vi "Controller - Fire Command.vi"(8 "error in (no error)":errorcluster, 9 "Data":variant, 10 "CMD":T1, 11 "View Model":T2) -> (0 "error out":errorcluster)   [LabVIEW 2017]
doc: "Generate command with parameters to Controller"
uses:
  View Model/Controls/View Model.ctl
  View Model/Controls/Shared Model.ctl
  Error Handler/Controls/Error Model.ctl
  Error Handler/Controls/Error Event.ctl
  Error Handler/Controls/Error Type.ctl
  Controls/Controller Model.ctl
  Controls/Controller Event.ctl
  Controls/Controller Command.ctl
  Controls/Controller Overhead.ctl
  Real-Time/RT Status.ctl
  Real-Time/RT Loop Status.ctl
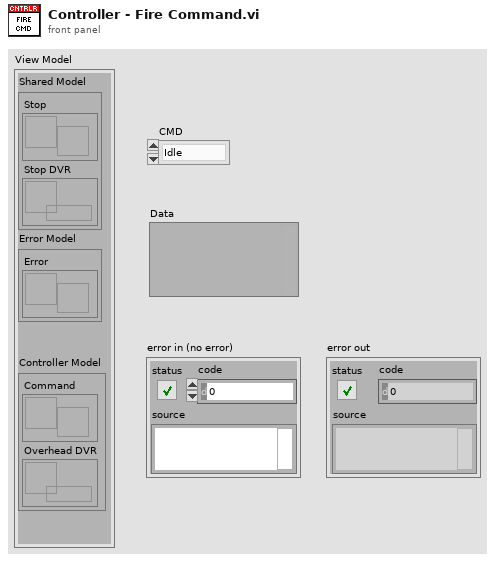
[diagram p1: front panel]
types:
  T1 = typedef "Controller Command.ctl" = enum16{"Idle", "Init", "Stop App", "Stop RT"}
  T2 = typedef "View Model.ctl" = cluster{"Shared Model":T3, "Error Model":T4, "Controller Model":T5}
  T3 = typedef "Shared Model.ctl" = cluster{"Stop":refnum<user-event>, "Stop DVR":refnum<data-value>}
  T4 = typedef "Error Model.ctl" = cluster{"Error":refnum<user-event>}
  T5 = typedef "Controller Model.ctl" = cluster{"Command":refnum<user-event>, "Overhead DVR":refnum<data-value>}
  T6 = typedef "Controller Event.ctl" = cluster{"CMD":T1, "Data":variant}
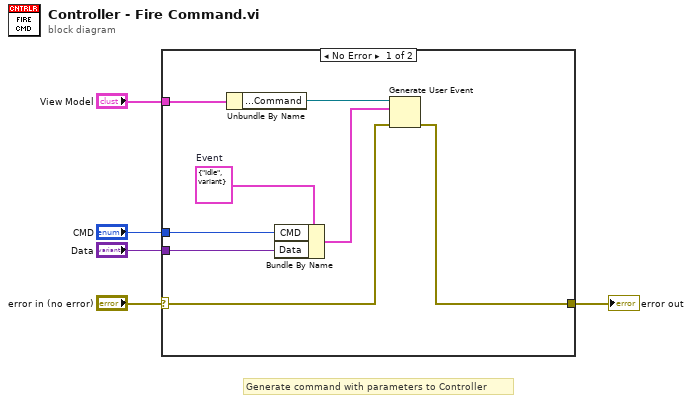
[diagram p0: block diagram]
diagram:
  # "Generate command with parameters to Controller"
  n1 = case shown="No Error" "error in (no error)" {
    selector: "error in (no error)" -> [w9 w14]
    tunnel: [w8 w14] -> w4
    tunnel: "View Model" -> [w13 _]
    tunnel: "Data" -> [w7 _]
    tunnel: "CMD" -> [w6 _]
    frame No Error {
      w11 = T6 {"CMD"=enum."Idle", "Data"=variant}  # Event
      n2 = Unbundle By Name(w13) -> ("Controller Model.Command"=w12:refnum<user-event>)
      n3 = Bundle By Name(cluster=w11, "CMD"=w6, "Data"=w7) -> (w10:T6)
      n4 = Generate User Event(user event=w12, event data cluster=w10, error in=w9) -> (error out=w8:errorcluster)  [unwired: 1 in, 1 out]
    }
    frame Error {
    }
  }
  "error out" <- w4
